vi "ListUserExperiments.vi"(10 "Search":string, 11 "Current user path":path) -> (3 "Sorted Array out":string[](array[string]))   [LabVIEW 2017]
uses:
  <userlib>/_OpenG.lib/file/file.llb/File Exists - Scalar__ogtk.vi
  <userlib>/_OpenG.lib/array/array.llb/Conditional Auto-Indexing Tunnel (String)__ogtk.vi
  <userlib>/_OpenG.lib/array/array.llb/Sort 1D Array (String)__ogtk.vi
  <vilib>/regexp/Match Regular Expression.xnode
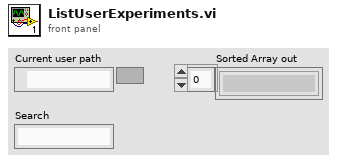
[diagram p1: front panel]
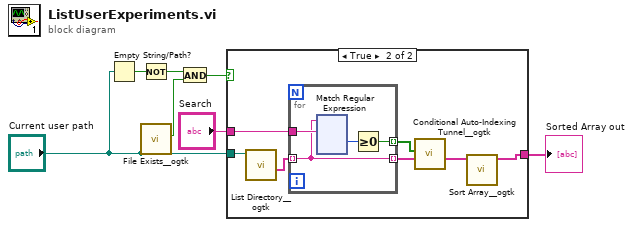
[diagram p0: block diagram]
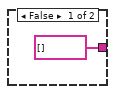
[diagram p2: hidden frame]
diagram:
  n1 = Empty String/Path?(string/path="Current user path") -> (empty?=w5:bool)
  n2 = Not(x=w5) -> (.not. x?=w3:bool)
  n3 = call-poly <userlib>:"File Exists__ogtk.vi"("file path"="Current user path") -> ("is directory"=w2:bool)  [unwired: 6 in, 1 out]
  n4 = And(x=w3, y=w2) -> (x .and. y?=w1:bool)
  n5 = case shown="True" w1 {
    tunnel: "Current user path" -> [_ w15]
    tunnel: [string[] [] ("Sorted Array out") w9] -> w6
    tunnel: "Search" -> [_ w14]
    frame False {
    }
    frame True {
      n6 = call <userlib>:"List Directory__ogtk.vi"("directory path"=w15) -> ("directory names"=w13:string[])  [unwired: 3 in, 3 out]
      n7 = for {
        tunnel: w14 -> [w19]
        tunnel: w13 -> [w16] mode=indexing
        tunnel: [w17] -> w11 mode=indexing
        tunnel: [w16] -> w12 mode=indexing
        n8 = xnode "Match Regular Expression"("input string"=w16, "regular expression"=w19) -> ("offset past match"=w18:i32)  [unwired: 4 in, 4 out]
        n9 = Greater Or Equal To 0?(x=w18) -> (x >= 0?=w17:bool)
      }
      n10 = call-poly <userlib>:"Conditional Auto-Indexing Tunnel__ogtk.vi"("Array in"=w12, "Elements to keep"=w11) -> ("Filtered Array out"=w10:string[])  [unwired: 5 in]
      n11 = call-poly <userlib>:"Sort Array__ogtk.vi"("Array in"=w10) -> ("Sorted Array out"=w9:string[])  [unwired: 9 in, 1 out]
    }
  }
  "Sorted Array out" <- w6
